vi "Logger 2.vi"(5 "output cluster":T1, 8 "RAW NAPEDY 2":T2, 9 "ON/OFF LOG":bool, 11 "path":path) -> ()   [LabVIEW 2015]
panel:
  in  "concatenated string 2":string="02:18:29,576;L1;L2;L3;P1;P2;P3;zapylenie;kierunek wiatru;predkosc wiatru;temp pkt rosy;PH;temp1;wilgotnosc;metan\r"
  out "concatenated string":string
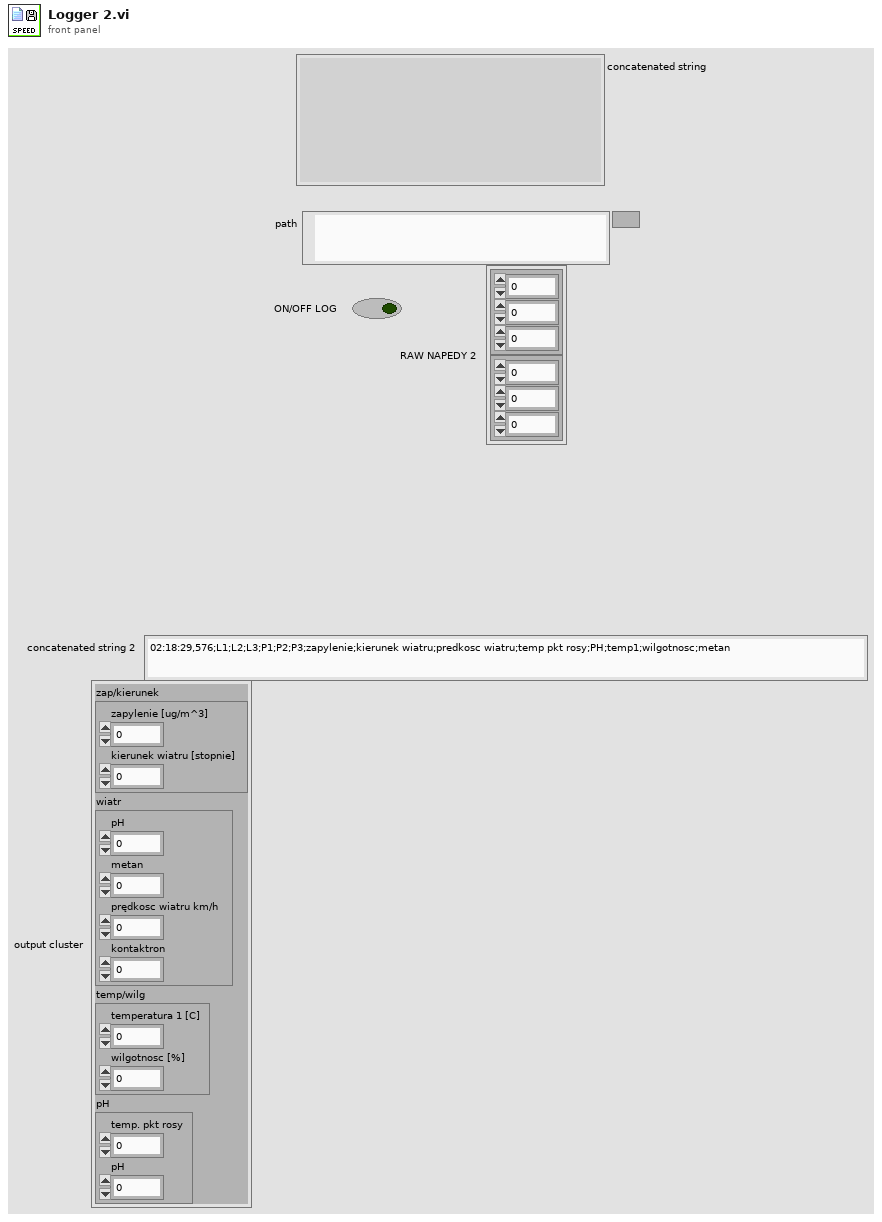
[diagram p1: front panel]
types:
  T1 = cluster{"zap/kierunek":cluster{"zapylenie [ug/m^3] ":sgl, "kierunek wiatru [stopnie]":sgl}, "wiatr":cluster{"pH":sgl, "metan":u8, "prędkosc wiatru km/h":u16, "kontaktron":u8}, "temp/wilg":cluster{"temperatura 1 [C]":sgl, "wilgotnosc [%]":sgl}, "pH":cluster{"temp. pkt rosy":sgl, "pH":sgl}}
  T2 = cluster{cluster{i16, i16, i16}, cluster{i16, i16, i16}}
  T3 = cluster{"zapylenie [ug/m^3] ":sgl, "kierunek wiatru [stopnie]":sgl}
  T4 = cluster{"pH":sgl, "metan":u8, "prędkosc wiatru km/h":u16, "kontaktron":u8}
  T5 = cluster{"temperatura 1 [C]":sgl, "wilgotnosc [%]":sgl}
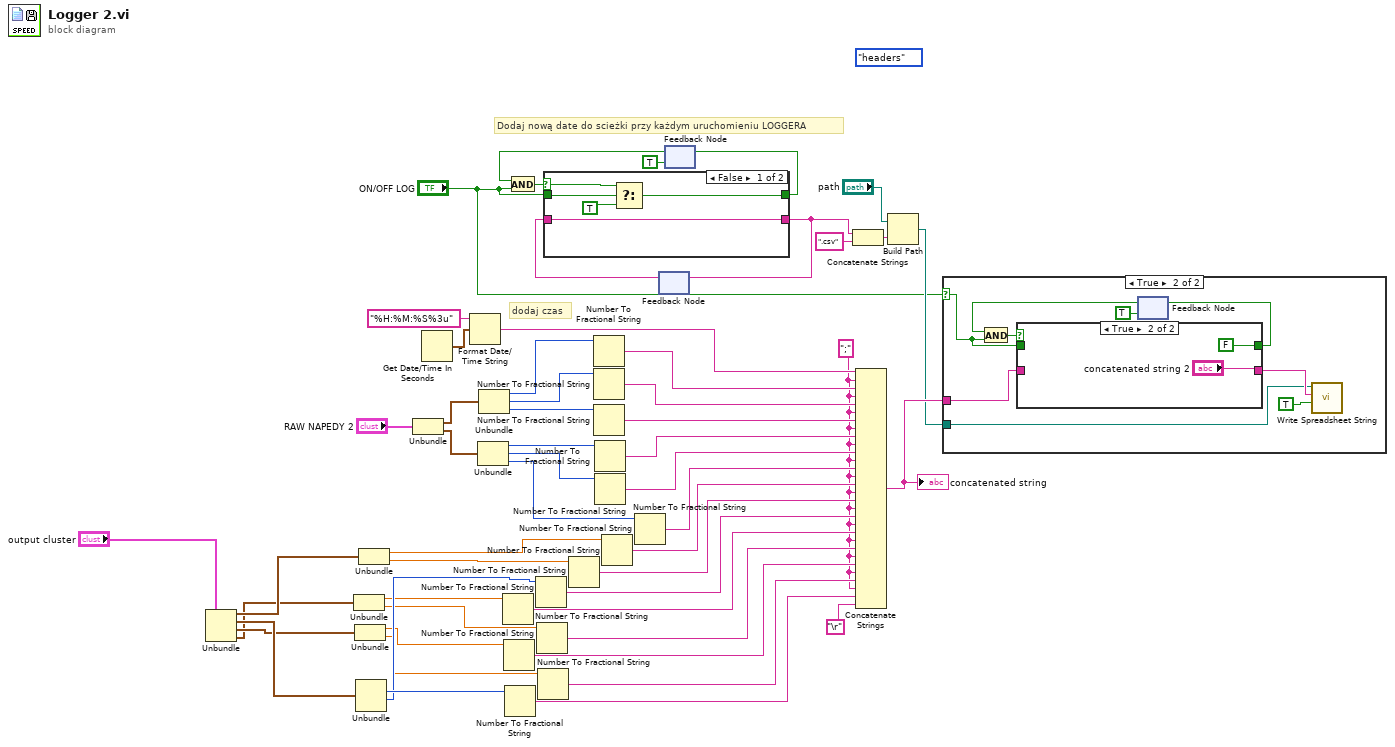
[diagram p0: block diagram]
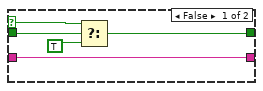
[diagram p3: hidden frame]
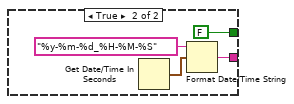
[diagram p4: hidden frame]
diagram:
  (unwired) enum16{"headers", "data"}."headers"
  w9 = ";" ("delimiter (\\t)")
  # "dodaj czas"
  # "Dodaj nową date do scieżki przy każdym uruchomieniu LOGGERA"
  n1 = Unbundle("output cluster") -> ("zap/kierunek"=w21:T3, "wiatr"=w23:T4, "temp/wilg"=w22:T5, "pH"=w7:cluster{"temp. pkt rosy":sgl, "pH":sgl})
  n2 = Unbundle(w7) -> ("temp. pkt rosy"=w4:sgl, "pH"=w3:sgl)
  n3 = Unbundle(w22) -> ("temperatura 1 [C]"=w2:sgl, "wilgotnosc [%]"=w1:sgl)
  n4 = Unbundle(w23) -> ("metan"=w6:u8, "prędkosc wiatru km/h"=w5:u16)  [unwired: 2 out]
  n5 = Unbundle(w21) -> ("zapylenie [ug/m^3]"=w20:sgl, "kierunek wiatru [stopnie]"=w19:sgl)
  n6 = Unbundle("RAW NAPEDY 2") -> (w42:cluster{i16, i16, i16}, w38:cluster{i16, i16, i16})
  n7 = Get Date/Time In Seconds() -> (seconds since 1Jan1904=w48:timestamp)
  n8 = Format Date/Time String(time format string (%c)="%H:%M:%S%3u", seconds (now)=w48) -> (date/time string=w47:string)  [unwired: 1 in]
  n9 = Unbundle(w38) -> (w37:i16, w36:i16, w35:i16)
  n10 = Unbundle(w42) -> (w41:i16, w40:i16, w39:i16)
  n11 = Number To Fractional String(number=w4) -> (F-format string=w15:string)  [unwired: 3 in]
  n12 = Number To Fractional String(number=w2) -> (F-format string=w13:string)  [unwired: 3 in]
  n13 = Number To Fractional String(number=w6) -> (F-format string=w11:string)  [unwired: 3 in]
  n14 = Number To Fractional String(number=w5) -> (F-format string=w16:string)  [unwired: 3 in]
  n15 = Number To Fractional String(number=w3) -> (F-format string=w14:string)  [unwired: 3 in]
  n16 = Number To Fractional String(number=w1) -> (F-format string=w12:string)  [unwired: 3 in]
  n17 = Number To Fractional String(number=w19) -> (F-format string=w17:string)  [unwired: 3 in]
  n18 = Number To Fractional String(number=w41) -> (F-format string=w46:string)  [unwired: 3 in]
  n19 = Number To Fractional String(number=w40) -> (F-format string=w45:string)  [unwired: 3 in]
  n20 = Number To Fractional String(number=w39) -> (F-format string=w44:string)  [unwired: 3 in]
  n21 = Number To Fractional String(number=w37) -> (F-format string=w51:string)  [unwired: 3 in]
  n22 = Number To Fractional String(number=w36) -> (F-format string=w52:string)  [unwired: 3 in]
  n23 = Number To Fractional String(number=w20) -> (F-format string=w18:string)  [unwired: 3 in]
  n24 = Number To Fractional String(number=w35) -> (F-format string=w53:string)  [unwired: 3 in]
  n25 = feedback #1() -> (w29:string)  [unwired: 1 in]
  n26 = feedback #2(TRUE) -> (w26:bool)
  n27 = And(x=w26, y="ON/OFF LOG") -> (x .and. y?=w25:bool)
  n28 = case shown="False" w25 {
    selector: w25 -> [w54 _]
    tunnel: [w58 w60] -> w30
    tunnel: [w57 FALSE] -> w28
    tunnel: w29 -> [w58 _]
    tunnel: "ON/OFF LOG" -> [w55 _]
    frame False {
      n29 = Select(t=w54, s=w55, f=TRUE) -> (s? t:f=w57:bool)
    }
    frame True {
      n30 = Get Date/Time In Seconds() -> (seconds since 1Jan1904=w62:timestamp)
      n31 = Format Date/Time String(time format string (%c)="%y-%m-%d_%H-%M-%S", seconds (now)=w62) -> (date/time string=w60:string)  [unwired: 1 in]
    }
  }
  n32 = feedback-in #1(w30) -> ()
  n33 = feedback-in #2(w28) -> ()
  n34 = Concatenate Strings(w30, ".csv" ("string")) -> (w34:string)
  n35 = Concatenate Strings(w47, w9, w46, w9, w45, w9, w44, w9, w51, w9, w52, w9, w53, w9, w18, w9, w17, w9, w16, w9, w15, w9, w14, w9, w13, w9, w12, w9, w11, "\r") -> (w50:string)
  "concatenated string" <- w50
  n36 = Build Path(base path="path", name or relative path=w34) -> (appended path=w31:path)
  n37 = case shown="True" "ON/OFF LOG" {
    selector: "ON/OFF LOG" -> [_ w67]
    tunnel: w50 -> [_ w64]
    tunnel: w31 -> [_ w63]
    frame False {
    }
    frame True {
      n38 = feedback #3(TRUE) -> (w70:bool)
      n39 = And(x=w70, y=w67) -> (x .and. y?=w71:bool)
      n40 = case shown="True" w71 {
        selector: w71 -> [w72 _]
        tunnel: [w76 "concatenated string 2"] -> w65
        tunnel: [w75 FALSE] -> w68
        tunnel: w64 -> [w76 _]
        tunnel: w67 -> [w73 _]
        frame False {
          n41 = Select(t=w72, s=w73, f=TRUE) -> (s? t:f=w75:bool)
        }
        frame True {
        }
      }
      n42 = feedback-in #3(w68) -> ()
      n43 = call <vilib>:"Write Spreadsheet String.vi"("append to file? (new file:F)"=TRUE, "spreadsheet string"=w65, "file path (dialog if empty)"=w63) -> ()  [unwired: 7 in, 2 out]
    }
  }
